vi "read analog HP.vi"(8 "error in (no error)":errorcluster, 11 "ID":i32) -> (0 "error out":errorcluster, 3 "Type Signal":T1={"DAQ Board Name"="DAQ_Simu1", "Analogicos Canales"=["DAQ_Simu1/ai1", "DAQ_Simu1/ai2"], "rate"=1000.0, "number of samples "=1000, "Tiempo"=100})   [LabVIEW 2020, in "Settings.lvlib"]
uses:
  Settings.lvlib
  typeSignal--cluster.ctl
  <vilib>/drjdpowell/SQLite Library/SQL Connection/Open (path).vi
  <vilib>/drjdpowell/SQLite Library/SQL Connection/Open (string).vi
  <vilib>/AdvancedString/Path To Command Line String.vi
  <vilib>/drjdpowell/SQLite Library/SQL Connection/Execute SQL (1D UTF-8).vi
  <vilib>/drjdpowell/SQLite Library/SQL Connection/Connection.lvclass
  <vilib>/drjdpowell/SQLite Library/SQLite.lvlib
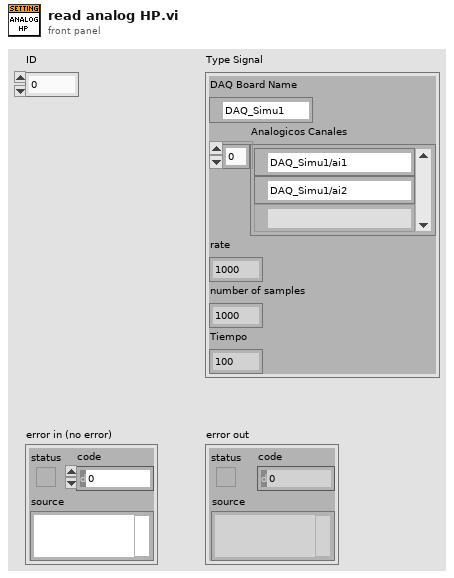
[diagram p1: front panel]
types:
  T1 = typedef "typeSignal--cluster.ctl" = cluster{"DAQ Board Name":tag, "Analogicos Canales":tag[], "rate":dbl, "number of samples ":i32, "Tiempo":i32}
  T2 = cluster{"Result Set (UTF-8)[0]":string, "Result Set (UTF-8)[1]":string, "Result Set (UTF-8)[2]":string, "Result Set (UTF-8)[3]":string, "Result Set (UTF-8)[4]":string, "Result Set (UTF-8)[5]":string, "Result Set (UTF-8)[6]":string, "Result Set (UTF-8)[7]":string, "Result Set (UTF-8)[8]":string}
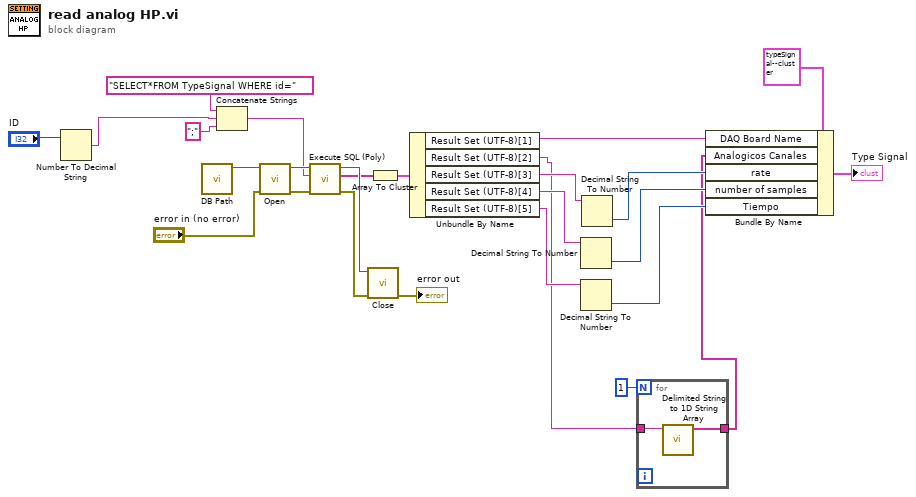
[diagram p0: block diagram]
diagram:
  n1 = Number To Decimal String(number="ID") -> (decimal integer string=w13:string)  [unwired: 1 in]
  n2 = call "DB Path.vi"() -> ("DB path"=w18:path)  [unwired: 11 in]
  n3 = Concatenate Strings("SELECT*FROM TypeSignal WHERE id=" ("SQL"), w13, ";" ("string")) -> (w15:string)
  n4 = call-poly <vilib>:"Open.vi"("error in (no error)"="error in (no error)", "db file"=w18) -> ("error out"=w26:errorcluster, "SQLite Connection"=w25:refnum<class "Connection.lvclass">)  [unwired: 8 in]
  n5 = call-poly <vilib>:"Execute SQL (Poly).vi"("error in (no error)"=w26, "SQL"=w15, "SQLite Connection in"=w25) -> ("error out"=w23:errorcluster, "Result Set (UTF-8)"=w19:string[], "SQLite Connection"=w24:refnum<class "Connection.lvclass">)  [unwired: 5 in, 1 out]
  n6 = call-dynamic "Close.vi"("error in (no error)"=w23, "SQLite Connection in"=w24) -> ("error out"=→"error out":errorcluster)  [unwired: 9 in]
  n7 = Array To Cluster(array=w19) -> (cluster=w20:T2)
  n8 = Unbundle By Name(w20) -> ("Result Set (UTF-8)[1]"=w9:string, "Result Set (UTF-8)[2]"=w2:string, "Result Set (UTF-8)[3]"=w8:string, "Result Set (UTF-8)[4]"=w7:string, "Result Set (UTF-8)[5]"=w6:string)
  n9 = Decimal String To Number(string=w7) -> (number=w11:i32)  [unwired: 2 in, 1 out]
  n10 = Decimal String To Number(string=w6) -> (number=w10:i32)  [unwired: 2 in, 1 out]
  n11 = Decimal String To Number(string=w8) -> (number=w12:i32)  [unwired: 2 in, 1 out]
  n12 = for {
    N: 1 -> [_]
    tunnel: [w28] -> w1
    tunnel: w2 -> [w27]
    n13 = call <vilib>:"Delimited String to 1D String Array.vi"("delimited string"=w27) -> ("string array"=w28:string[])  [unwired: 10 in]
  }
  n14 = Bundle By Name(cluster=T1 {"DAQ Board Name"="DAQ_Simu1", "Analogicos Canales"=["DAQ_Simu1/ai0", "\t", "\t", "\t", "\t", "\t", "\t", "\t"], "rate"=15.0, "number of samples "=100, "Tiempo"=4} ("Type Signal"), "DAQ Board Name"=w9, "Analogicos Canales"=w1, "rate"=w12, "number of samples"=w11, "Tiempo"=w10) -> (→"Type Signal":T1)
